vi "Read Self Actor.vi"(11 "Read Self Actor in":refnum<class "Read Self Actor.lvclass">) -> (2 "Self Actor":refnum<class "LVCAM.lvclass">)   [LabVIEW 2021, in "LVCAM.lvlib" / "Read Self Actor.lvclass"]
uses:
  Read Self Actor.lvclass
  LVCAM/LVCAM.lvclass
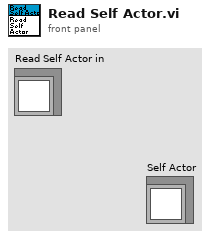
[diagram p1: front panel]
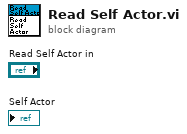
[diagram p0: block diagram]
diagram:
